vi "Main.vi"() -> ()   [LabVIEW 2020]
doc: "This template is for the Queued Message Handler design pattern.\n\nThe Event Handling Loop generates messages based on user interface actions.\n\nThe Message Handling Loop processes messages generated by the Event Handling Loop, or by other messages. The messages are string values, so new messages can be added easily to the Message Cases case structure in the Message Handling Loop. Each message cluster can also provide an optional value for Message Data, which is a variant that can be converted to whatever message-specific data is required."
uses:
  controls/UI Data.ctl
  game/Direction.ctl
  game/New Value Mode.ctl
  game/Game Status.ctl
  support/Message Queue/Enqueue Message (Single).vi
  <vilib>/Utility/error.llb/Error Cluster From Error Code.vi
  <vilib>/ErrorRing/Error Ring.xnode
  support/Message Queue/Message Queue.lvlib
  support/User Event - Stop/User Event - Stop.lvlib
  game/Game.lvlib
panel:
  out "Board":u8[][](array[ring])
  out "Score":string
  in  "Exit":bool
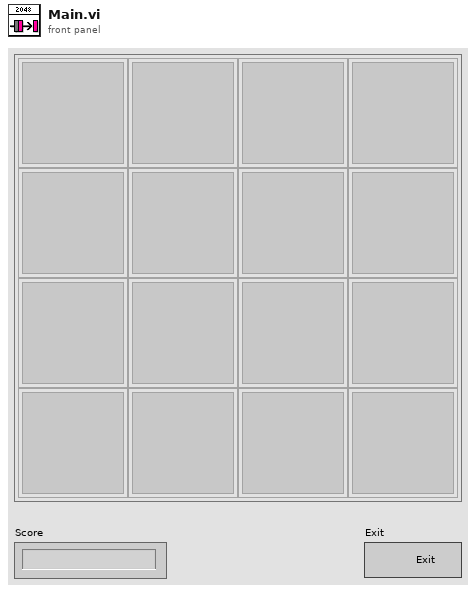
[diagram p1: front panel]
types:
  T1 = typedef "UI Data.ctl" = cluster{"Score":i32, "Board Array":u8[][], "Board":refnum<vi>}
  T2 = typedef "Message Queue.lvlib/All Message Queues.ctl" = cluster{"UI":refnum<queue>}
  T3 = typedef "Direction.ctl" = enum16{"Up", "Down", "Left", "Right"}
  T4 = typedef "eventvkey.ctl" = enum16{"ASCII", "Enter", "Return", "Shift", "Ctrl", "Alt", "Cmd", "Opt", "Caps", "NumLock", "Clear", "Break", "Up", "Down", "Left", "Right", "Insert", "Delete", "Home", "End", "PageUp", "PageDown", "Escape", "Help", "Pause", "ScrollLock", "F1", "F2", "F3", "F4", "F5", "F6", "F7", "F8", "F9", "F10", "F11", "F12", "F13", "F14", "F15", "F16", "F17", "F18", "F19", "F20", "F21", "F22", "F23", "F24", "Play", "VolumeUp", "VolumeDown", "Mute", "Two Byte Char"}
  T5 = typedef "New Value Mode.ctl" = enum16{"In Game", "Initial Game"}
  T6 = typedef "Game Status.ctl" = enum16{"Winnig", "Game Over", "Continute"}
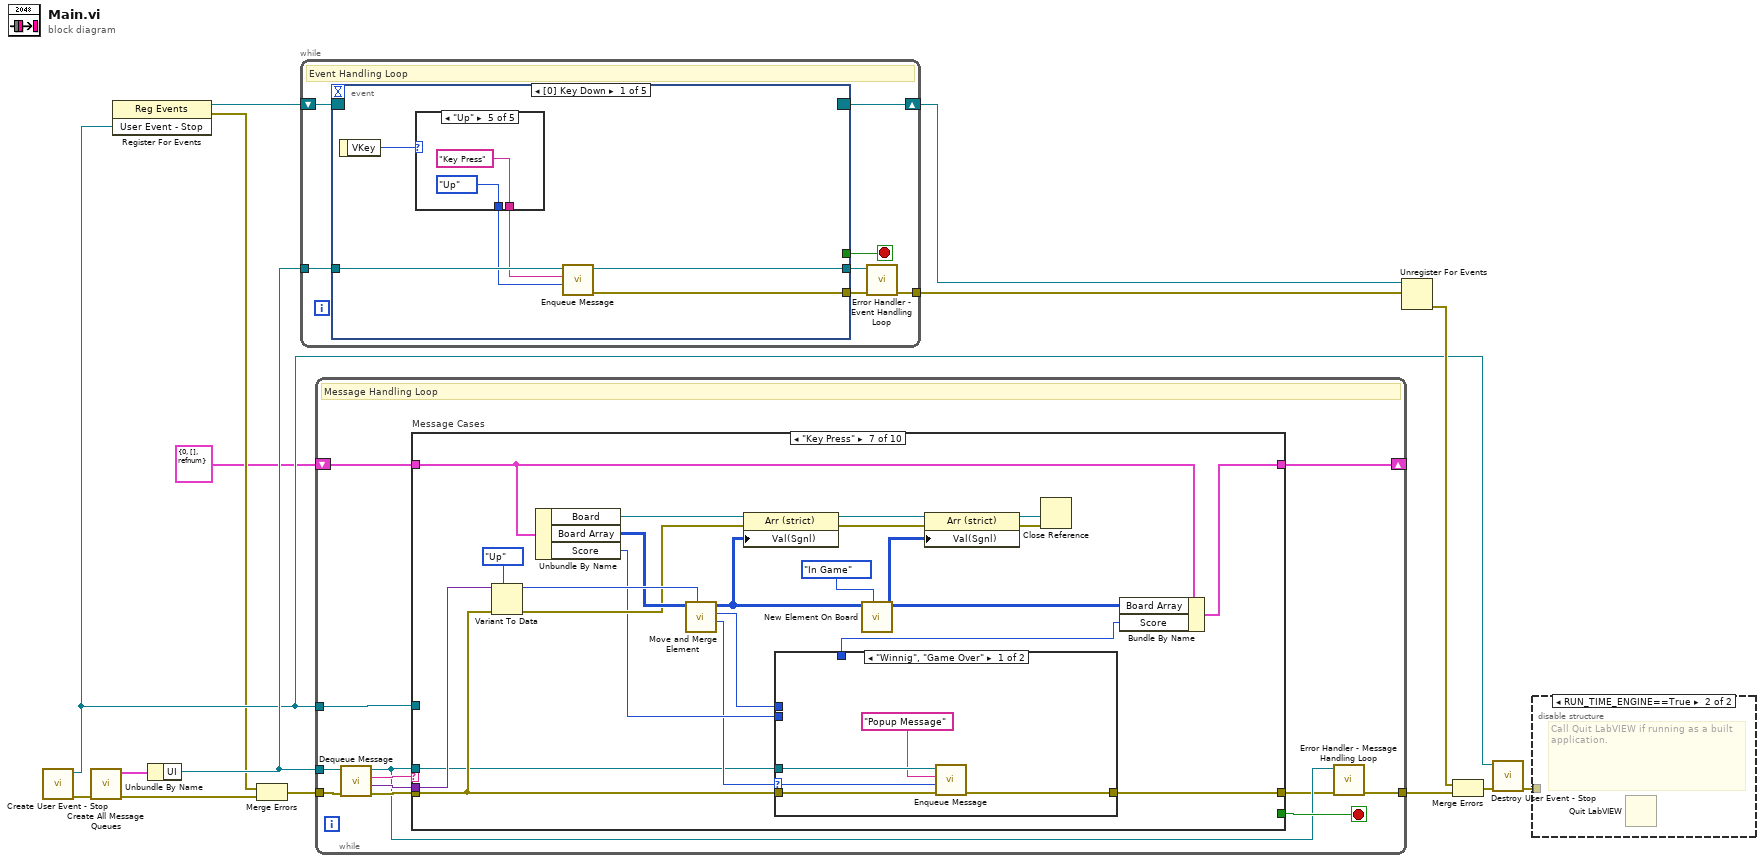
[diagram p0: block diagram]
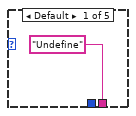
[diagram p3: hidden frame]
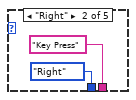
[diagram p4: hidden frame]
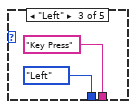
[diagram p5: hidden frame]
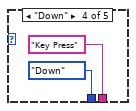
[diagram p6: hidden frame]
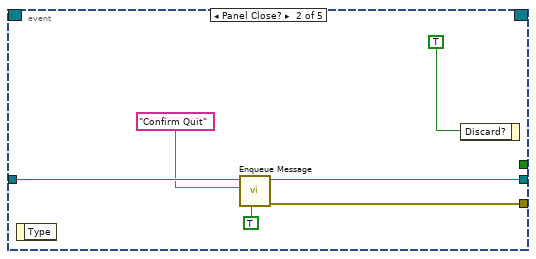
[diagram p7: hidden frame]
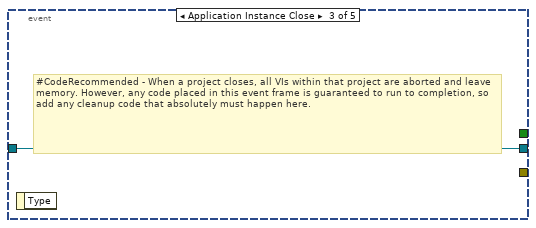
[diagram p8: hidden frame]
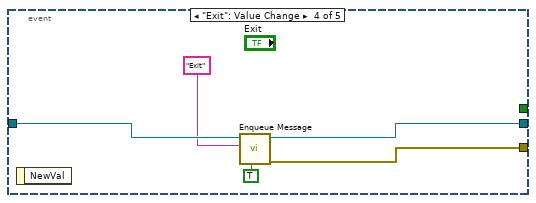
[diagram p9: hidden frame]
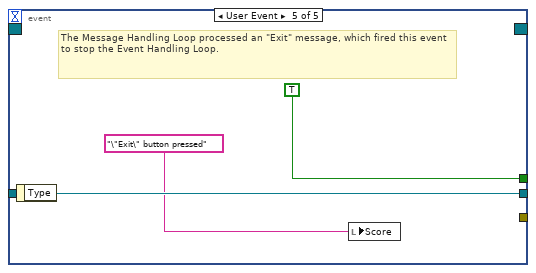
[diagram p10: hidden frame]
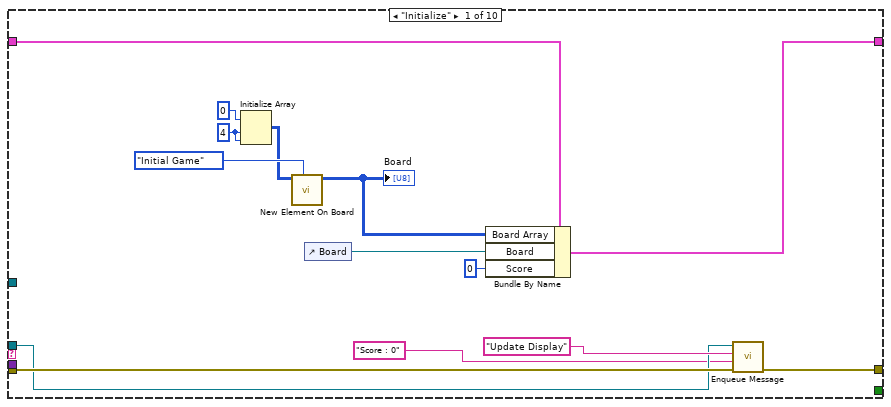
[diagram p11: hidden frame]
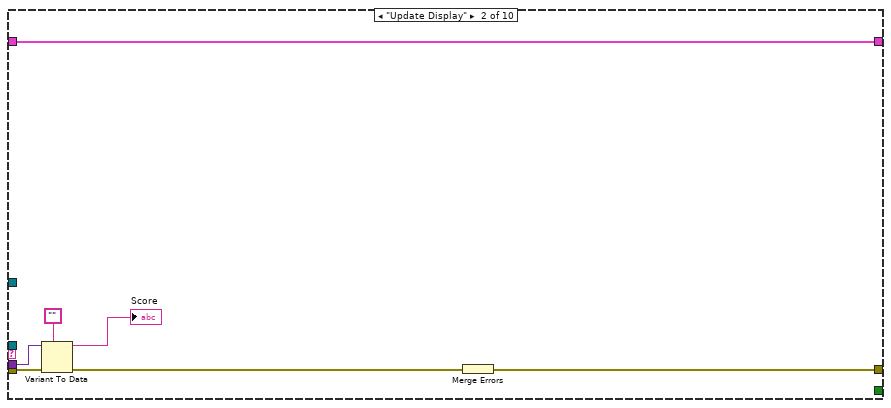
[diagram p12: hidden frame]
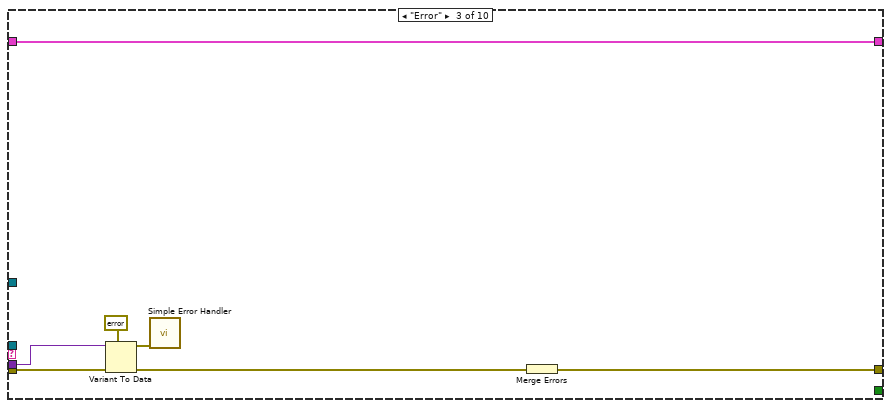
[diagram p13: hidden frame]
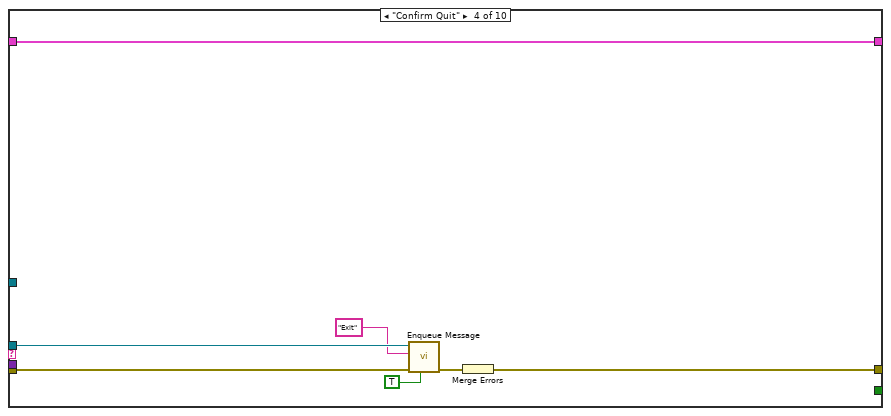
[diagram p14: hidden frame]
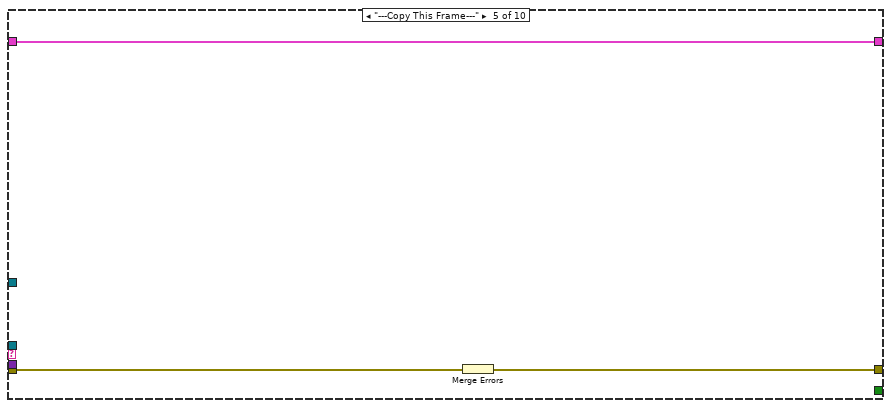
[diagram p15: hidden frame]
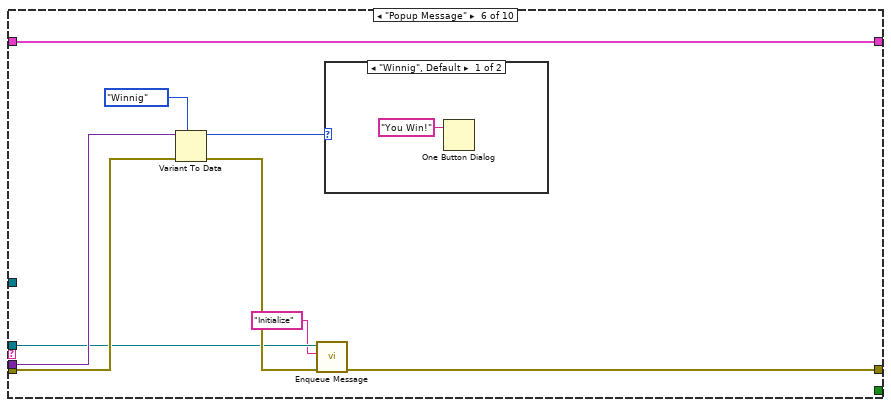
[diagram p16: hidden frame]
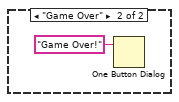
[diagram p17: hidden frame]
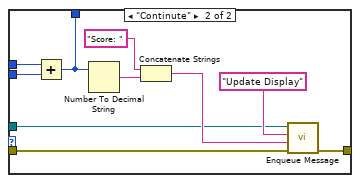
[diagram p18: hidden frame]
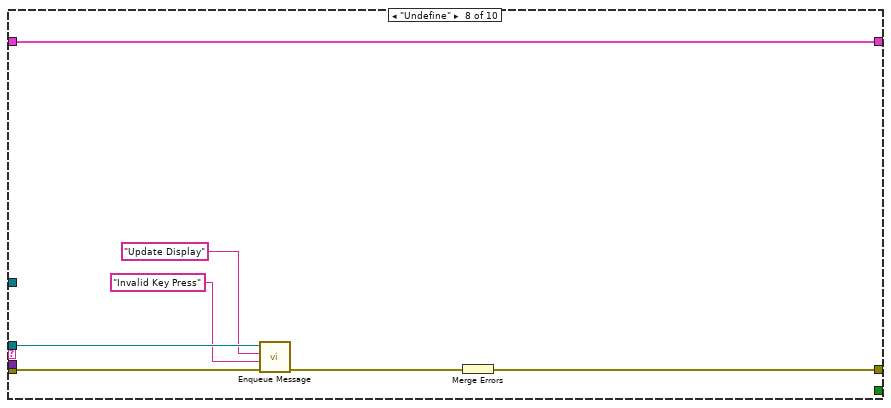
[diagram p19: hidden frame]
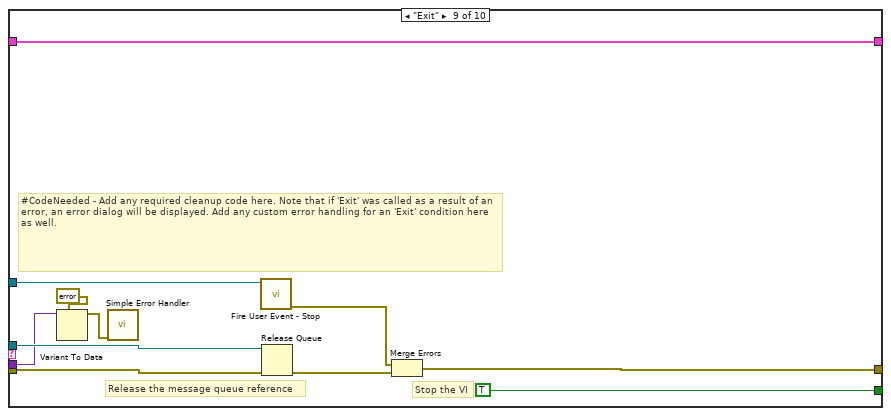
[diagram p20: hidden frame]
diagram:
  n1 = call "Create User Event - Stop.vi"() -> ("error out"=w11:errorcluster, "User Event - Stop"=w4:refnum<user-event>)  [unwired: 10 in]
  n2 = call "Create All Message Queues.vi"("error in (no error)"=w11) -> ("error out"=w15:errorcluster, "Message Queues out"=w14:T2)  [unwired: 9 in]
  n3 = register-events(w4) -> (reference out=w5:refnum<event-registration>, error out=w2:errorcluster)  [unwired: 2 in]
  n4 = Unbundle By Name(w14) -> ("UI"=w12:refnum<queue>)
  n5 = Merge Errors(w2, w15) -> (w3:errorcluster)
  n6 = while {
    tunnel: w12 -> [w22]
    shift-right: [w20] -> w8
    shift-left: w5 -> [w21]
    tunnel: [w16] -> w6
    stop <- w18 stop-if-true
    # "Event Handling Loop"
    n7 = event shown="[0] Key Down" {
      selector: w21 -> [_ _ _ _ _]
      dyn-events: [_ _ _ _ _] -> w20
      timeout: _ -> [_ _ _ _ _]
      tunnel: [_ _ _ _ TRUE ("Discard?")] -> w18
      tunnel: w22 -> [w28 w42 w44 w49 w52]
      tunnel: [w26 w41 _ w48 _] -> w19
      tunnel: [w27 w40 w44 w47 w52] -> w17
      event Key Down {
        n8 = event-data() -> ("VKey"=w23:T4)  [unwired: 1 in]
        n9 = case shown="\"Up\"" w23 {
          tunnel: ["Undefine" ("Message") "Key Press" ("Message") "Key Press" ("Message") "Key Press" ("Message") "Key Press" ("Message")] -> w25
          tunnel: [_ Direction."Right" ("Direction") Direction."Left" ("Direction") Direction."Down" ("Direction") Direction."Up" ("Direction")] -> w24
          frame Default {
          }
          frame "Right" {
          }
          frame "Left" {
          }
          frame "Down" {
          }
          frame "Up" {
          }
        }
        n10 = call-poly "Enqueue Message.vi"("Message Data"=w24, "Message"=w25, "Message Queue"=w28) -> ("error out"=w26:errorcluster, "dup Message Queue"=w27:refnum<queue>)  [unwired: 7 in]
      }
      event Panel Close? {
        n11 = event-data() -> ()  [unwired: 1 in, 1 out]
        n12 = call-poly "Enqueue Message.vi"("Priority Message? (F)"=TRUE, "Message"="Confirm Quit", "Message Queue"=w42) -> ("error out"=w41:errorcluster, "dup Message Queue"=w40:refnum<queue>)  [unwired: 7 in]
        n13 = event-data("Discard?"=TRUE) -> ()  [unwired: 1 in, 1 out]
      }
      event Application Instance Close {
        # "#CodeRecommended - When a project closes, all VIs within that project are aborted and leave memory. However, any code placed in this event frame is guaranteed to run to completion, so add any cleanup code that absolutely must happen here."
        n14 = event-data() -> ()  [unwired: 1 in, 1 out]
      }
      event "Exit": Value Change {
        n15 = event-data() -> ()  [unwired: 1 in, 1 out]
        n16 = call-poly "Enqueue Message.vi"("Priority Message? (F)"=TRUE, "Message"="Exit", "Message Queue"=w49) -> ("error out"=w48:errorcluster, "dup Message Queue"=w47:refnum<queue>)  [unwired: 7 in]
      }
      event User Event {
        # "The Message Handling Loop processed an \"Exit\" message, which fired this event to stop the Event Handling Loop."
        n17 = event-data() -> ()  [unwired: 1 in, 1 out]
        n18 = local write "Score"("\"Exit\" button pressed" ("VI Stopped")) -> ()
      }
    }
    n19 = call "Error Handler - Event Handling Loop.vi"("error in (no error)"=w19, "Message Queue"=w17) -> ("dup error in"=w16:errorcluster)  [unwired: 8 in, 1 out]
  }
  n20 = while {
    tunnel: w12 -> [w56]
    shift-right: [w63] -> _
    shift-left: T1 {"Score"=0, "Board Array"=[], "Board"=refnum} ("UI Data") -> [w64]
    tunnel: w4 -> [w61]
    tunnel: w3 -> [w60]
    tunnel: [w54] -> w13
    stop <- w62 stop-if-true
    # "Message Handling Loop"
    n21 = call "Dequeue Message.vi"("error in (no error)"=w60, "Message Queue"=w56) -> ("error out"=w59:errorcluster, "Message Data"=w57:variant, "Message"=w58:string, "dup Message Queue"=w55:refnum<queue>)  [unwired: 6 in]
    n22 = case "Message Cases" shown="\"Key Press\"" w58 {
      selector: w58 -> [_ _ _ _ _ _ _ _ _ w169]
      tunnel: w55 -> [w73 _ _ w95 _ w105 w115 w153 w168 _]
      tunnel: w59 -> [w77 w83 w92 w99 w102 w110 w117 w155 w161 _]
      tunnel: [w78 w84 w86 w97 w100 w106 w116 w156 w164 w170] -> w53
      tunnel: w64 -> [w76 w85 w91 w98 w101 w111 w130 w157 w167 w171]
      tunnel: [w75 w85 w91 w98 w101 w111 w131 w157 w167 w171] -> w63
      tunnel: [_ _ _ _ _ _ _ _ TRUE _] -> w62
      tunnel: w57 -> [_ w82 w90 _ _ w108 w135 _ w158 _]
      tunnel: w61 -> [_ _ _ _ _ _ _ _ w163 _]
      frame "Initialize" {
        w70 = 4 ("dimension size")
        # "Initialize - All initialization work should take place in this message, since other loops can potentially enqueue messages that execute immediately after this one."
        n23 = Initialize Array(u8 0, w70, w70) -> (w67:u8[][])
        n24 = call "New Element On Board.vi"("New Value Mode"=New_Value_Mode."Initial Game", "Board Array"=w67) -> ("Board Array"=w66:u8[][])  [unwired: 9 in]
        "Board" <- w66
        n25 = control-ref of="Board"() -> (w68:refnum<vi>)
        n26 = Bundle By Name(cluster=w76, "Board Array"=w66, "Board"=w68, "Score"=0) -> (w75:T1)
        n27 = call-poly "Enqueue Message.vi"("error in (no error)"=w77, "Message Data"="Score : 0" ("Initial Message"), "Message"="Update Display", "Message Queue"=w73) -> ("error out"=w78:errorcluster)  [unwired: 6 in, 1 out]
      }
      frame "Update Display" {
        # "Update Display - Convert the message data to a string to display in the Data Display indicator."
        n28 = Variant To Data(error in=w83, type="", Variant=w82) -> (data=→"Score":string, error out=w80:errorcluster)
        n29 = Merge Errors(w80) -> (w84:errorcluster)
      }
      frame "Error" {
        # "Error - Display an error dialog. This message is sent by the \"Error Handler\" VIs at the end of other loops in this application."
        n30 = Variant To Data(error in=w92, type=errorcluster {"status"=FALSE, "code"=0, "source"=""} ("error constant"), Variant=w90) -> (data=w88:errorcluster, error out=w87:errorcluster)
        n31 = call <vilib>:"Simple Error Handler.vi"("error in (no error)"=w88) -> ()  [unwired: 4 in, 5 out]
        n32 = Merge Errors(w87) -> (w86:errorcluster)
      }
      frame "Confirm Quit" {
        # "Confirm Quit - Message that can confirm whether or not the user wants to exit the application."
        n33 = call-poly "Enqueue Message.vi"("Priority Message? (F)"=TRUE, "error in (no error)"=w99, "Message"="Exit", "Message Queue"=w95) -> ("error out"=w96:errorcluster)  [unwired: 6 in, 1 out]
        n34 = Merge Errors(w96) -> (w97:errorcluster)
      }
      frame "---Copy This Frame---" {
        # "Duplicate this frame when creating new messages.  Change this comment in the duplicated frame to describe this message."
        n35 = Merge Errors(w102) -> (w100:errorcluster)
      }
      frame "Popup Message" {
        # "Duplicate this frame when creating new messages.  Change this comment in the duplicated frame to describe this message."
        n36 = Variant To Data(error in=w110, type=Game_Status."Winnig" ("Game Status"), Variant=w108) -> (data=w104:T6, error out=w107:errorcluster)
        n37 = call-poly "Enqueue Message.vi"("error in (no error)"=w107, "Message"="Initialize", "Message Queue"=w105) -> ("error out"=w106:errorcluster)  [unwired: 7 in, 1 out]
        n38 = case shown="\"Winnig\", Default" w104 {
          frame "Winnig", Default {
            n39 = One Button Dialog(message="You Win!") -> ()  [unwired: 1 in, 1 out]
          }
          frame "Game Over" {
            n40 = One Button Dialog(message="Game Over!") -> ()  [unwired: 1 in, 1 out]
          }
        }
      }
      frame "Key Press" {
        # "Duplicate this frame when creating new messages.  Change this comment in the duplicated frame to describe this message."
        n41 = Variant To Data(error in=w117, type=Direction."Up" ("Direction"), Variant=w135) -> (data=w133:T3, error out=w121:errorcluster)
        n42 = Unbundle By Name(w130) -> ("Board"=w129:refnum<vi>, "Board Array"=w126:u8[][], "Score"=w120:i32)
        n43 = call "Move and Merge Element.vi"("Direction"=w133, "Board Array"=w126) -> ("Game Status"=w118:T6, "Score"=w119:i32, "Board Array"=w125:u8[][])  [unwired: 7 in]
        n44 = property class="Arr (strict)"(reference=w129, error in=w121, "Val(Sgnl)"=w125) -> (reference out=w128:refnum<vi>, error out=w127:errorcluster)
        n45 = case shown="\"Winnig\", \"Game Over\"" w118 {
          selector: w118 -> [w136 _]
          tunnel: w120 -> [_ w146]
          tunnel: w119 -> [_ w145]
          tunnel: w117 -> [w140 w144]
          tunnel: [w139 w143] -> w116
          tunnel: w115 -> [w138 w142]
          tunnel: [_ w141] -> w114
          frame "Winnig", "Game Over" {
            n46 = call-poly "Enqueue Message.vi"("error in (no error)"=w140, "Message Data"=w136, "Message"="Popup Message", "Message Queue"=w138) -> ("error out"=w139:errorcluster)  [unwired: 6 in, 1 out]
          }
          frame "Continute" {
            n47 = Add(x=w145, y=w146) -> (x+y=w141:i32)
            n48 = Number To Decimal String(number=w141) -> (decimal integer string=w148:string)  [unwired: 1 in]
            n49 = Concatenate Strings("Score: " ("string"), w148) -> (w147:string)
            n50 = call-poly "Enqueue Message.vi"("error in (no error)"=w144, "Message Data"=w147, "Message"="Update Display", "Message Queue"=w142) -> ("error out"=w143:errorcluster)  [unwired: 6 in, 1 out]
          }
        }
        n51 = call "New Element On Board.vi"("New Value Mode"=New_Value_Mode."In Game", "Board Array"=w125) -> ("Board Array"=w124:u8[][])  [unwired: 9 in]
        n52 = property class="Arr (strict)"(reference=w128, error in=w127, "Val(Sgnl)"=w124) -> (reference out=w123:refnum<vi>, error out=w122:errorcluster)
        n53 = Close Reference(reference=w123, error in (no error)=w122) -> ()  [unwired: 1 out]
        n54 = Bundle By Name(cluster=w130, "Board Array"=w124, "Score"=w114) -> (w131:T1)
      }
      frame "Undefine" {
        # "Duplicate this frame when creating new messages.  Change this comment in the duplicated frame to describe this message."
        n55 = call-poly "Enqueue Message.vi"("error in (no error)"=w155, "Message Data"="Invalid Key Press" ("Message"), "Message"="Update Display", "Message Queue"=w153) -> ("error out"=w154:errorcluster)  [unwired: 6 in, 1 out]
        n56 = Merge Errors(w154) -> (w156:errorcluster)
      }
      frame "Exit" {
        # "Stop the VI"
        # "Release the message queue reference"
        # "#CodeNeeded - Add any required cleanup code here. Note that if 'Exit' was called as a result of an error, an error dialog will be displayed. Add any custom error handling for an 'Exit' condition here as well."
        # "Exit - Exit the application."
        n57 = Variant To Data(type=errorcluster {"status"=FALSE, "code"=0, "source"=""} ("error constant"), Variant=w158) -> (data=w159:errorcluster)  [unwired: 1 in, 1 out]
        n58 = call <vilib>:"Simple Error Handler.vi"("error in (no error)"=w159) -> ()  [unwired: 4 in, 5 out]
        n59 = call "Fire User Event - Stop.vi"("User Event - Stop"=w163) -> ("error out"=w162:errorcluster)  [unwired: 10 in]
        n60 = Release Queue(queue=w168, error in (no error)=w161) -> (error out=w165:errorcluster)  [unwired: 1 in, 2 out]
        n61 = Merge Errors(w162, w165) -> (w164:errorcluster)
      }
      frame Default {
        # "'Default' case only runs if there is a message that isn't defined in any of the other cases.  Output a programming error."
        n62 = xnode "Error Ring"("parameter 0"=w169) -> ("error out"=w170:errorcluster)
      }
    }
    n63 = call "Error Handler - Message Handling Loop.vi"("error in (no error)"=w53, "Message Queue"=w55) -> ("dup error in"=w54:errorcluster)  [unwired: 8 in, 1 out]
  }
  n64 = Unregister For Events(event registration refnum=w8, error in=w6) -> (error out=w9:errorcluster)
  n65 = Merge Errors(w9, w13) -> (w10:errorcluster)
  n66 = call "Destroy User Event - Stop.vi"("error in (no error)"=w10, "User Event - Stop"=w4) -> ("error out"=w7:errorcluster)  [unwired: 9 in]
  n67 = disable-structure shown="RUN_TIME_ENGINE==True" {
    disable-tunnel: w7 -> [_ _]
    frame condition #0 (active) {
    }
    frame condition #1 {
      # "Call Quit LabVIEW if running as a built application."
      n68 = Quit LabVIEW() -> ()  [unwired: 1 in]
    }
  }
